vi "Get Coefficient Caps.vi"(0 "Session Handle":T1, 11 "error in (no error)":errorcluster) -> (4 "Session Handle Out":T1, 6 "Ki Error":u16, 8 "Kd Error":u16, 10 "Max Cap":u16, 15 "error out":errorcluster)   [LabVIEW 2015, in "Peltier.lvclass"]
uses:
  Peltier.lvclass
  Typedefs/Session Handle.ctl
  PAS/PAS.lvclass
panel:
  out "Success?":bool
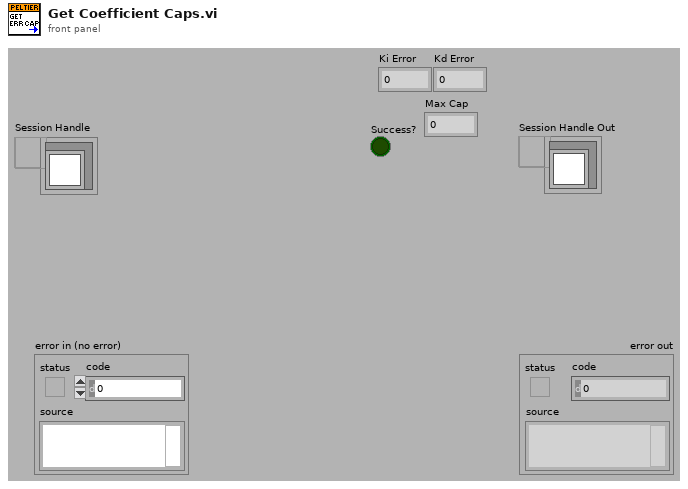
[diagram p1: front panel]
types:
  T1 = typedef "Peltier.lvclass/Session Handle.ctl" = refnum<data-value>
  T2 = typedef "XNET Frame CAN.ctl" = cluster{"timestamp":timestamp, "payload":u8[], "identifier":u32, "type":T3, "extended?":bool, "echo?":bool}
  T3 = typedef "XNET Frame Type CAN.ctl" = u8
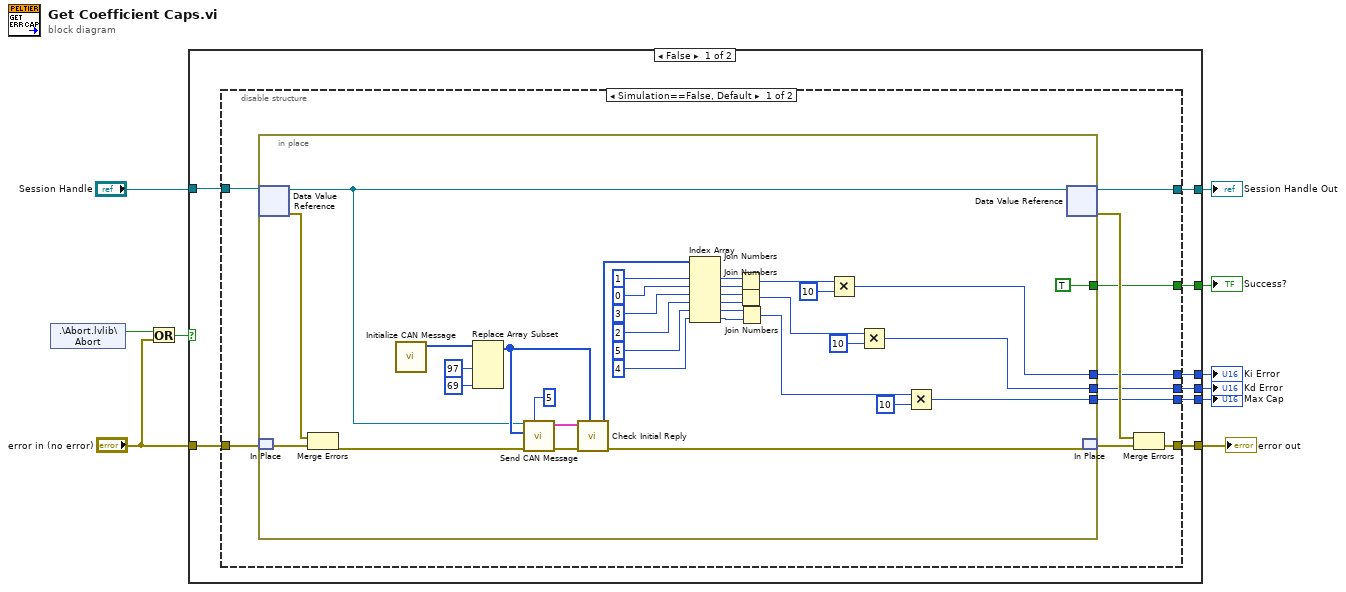
[diagram p0: block diagram]
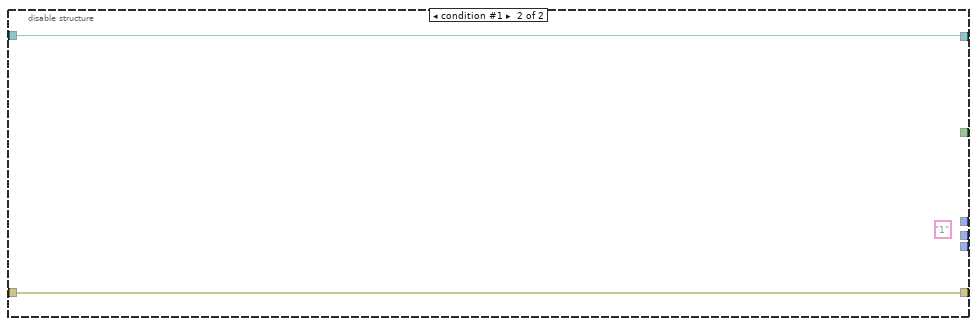
[diagram p2: hidden frame]
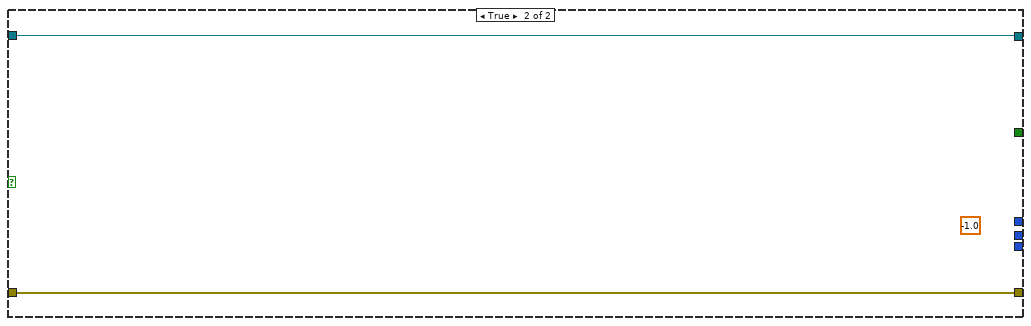
[diagram p3: hidden frame]
diagram:
  n1 = shared-variable ".\\Abort.lvlib\\Abort"() -> (w9:bool)  [unwired: 1 in, 1 out]
  n2 = Or(x=w9, y="error in (no error)") -> (x .or. y?=w7:bool)
  n3 = case shown="False" w7 {
    tunnel: [w18 w67] -> w5
    tunnel: [w17 w66] -> w10
    tunnel: "Session Handle" -> [w16 w67]
    tunnel: "error in (no error)" -> [w15 w66]
    tunnel: [w14 _] -> w4
    tunnel: [w13 _] -> w3
    tunnel: [w12 _] -> w2
    tunnel: [w11 _] -> w1
    frame False {
      n4 = disable-structure shown="Simulation==False, Default" {
        disable-tunnel: [w28 w65] -> w18
        disable-tunnel: [w25 w64] -> w17
        disable-tunnel: w16 -> [w24 w65]
        disable-tunnel: w15 -> [w23 w64]
        disable-tunnel: [w22 _] -> w14
        disable-tunnel: [w21 _] -> w13
        disable-tunnel: [w20 _] -> w12
        disable-tunnel: [w19 _] -> w11
        frame condition #0 (active) {
          n5 = in-place {
            in-place-border: [TRUE] -> w22
            in-place-border: [w38] -> w21
            in-place-border: [w32] -> w20
            in-place-border: [w31] -> w19
            n6 = in-place-dvr #1(w24) -> (w55:refnum<class "Peltier.lvclass">, w60:errorcluster)
            n7 = in-place-match #2(w23) -> (w59:errorcluster)
            n8 = Merge Errors(w60, w59) -> (w54:errorcluster)
            n9 = call "Initialize CAN Message.vi"() -> ("Initial Payload"=w62:u8[])  [unwired: 11 in]
            n10 = Replace Array Subset(array=w62, new element #1=u8 97 ("new element/subarray"), new element #2=u8 69 ("new element/subarray")) -> (w58:u8[])  [unwired: 2 in]
            n11 = call "Send CAN Message.vi"("Number of Retries"=5, "error in (no error)"=w54, "payload"=w58, "Peltier In"=w55) -> ("error out"=w30:errorcluster, "Reply"=w56:T2[])  [unwired: 5 in, 1 out]
            n12 = call "Check Initial Reply.vi"("Write Message"=w58, "error in (no error)"=w30, "Reply"=w56) -> ("error out"=w29:errorcluster, "Data Packet"=w61:u8[])  [unwired: 5 in, 2 out]
            n13 = Index Array(array=w61, index #1=1 ("index"), index #2=0 ("index"), index #3=3 ("index"), index #4=2 ("index"), index #5=5 ("index"), index #6=4 ("index")) -> (element #1=w44:u8, element #2=w45:u8, element #3=w42:u8, element #4=w41:u8, element #5=w40:u8, element #6=w39:u8)
            n14 = Join Numbers(hi=w44, lo=w45) -> ((hi.lo)=w43:u16)
            n15 = Join Numbers(hi=w42, lo=w41) -> ((hi.lo)=w35:u16)
            n16 = Join Numbers(hi=w40, lo=w39) -> ((hi.lo)=w33:u16)
            n17 = Multiply(x=w43, y=u16 10) -> (x*y=w38:u16)
            n18 = Multiply(x=w35, y=u16 10) -> (x*y=w32:u16)
            n19 = Multiply(x=w33, y=u16 10) -> (x*y=w31:u16)
            n20 = in-place-dvr #1(w55) -> (w28:T1, w26:errorcluster)
            n21 = in-place-match #2(w29) -> (w27:errorcluster)
          }
          n22 = Merge Errors(w26, w27) -> (w25:errorcluster)
        }
        frame condition #1 {
          (unwired) "1"
        }
      }
    }
    frame True {
      (unwired) -1.0
    }
  }
  "error out" <- w10
  "Success?" <- w4
  "Session Handle Out" <- w5
  "Ki Error" <- w3
  "Kd Error" <- w2
  "Max Cap" <- w1
